vi "lab #5 (displaying cos and sine wave continuously).vi"() -> ()   [LabVIEW 2016]
panel:
  out "Waveform Graph":dynamicdata(graph)
  in  "Phase":dbl
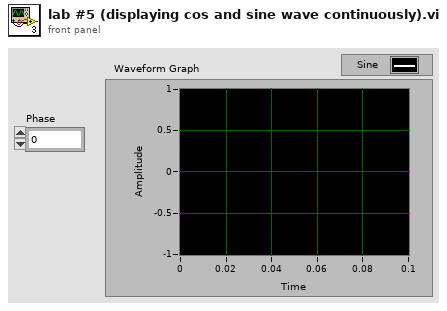
[diagram p1: front panel]
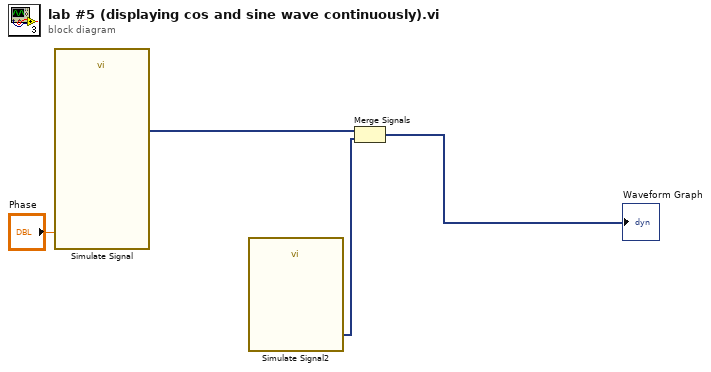
[diagram p0: block diagram]
diagram:
  n1 = call "Simulate Signal"("Phase"="Phase") -> ("Sine"=w4:dynamicdata)  [unwired: 13 in, 1 out]
  n2 = call "Simulate Signal2"() -> ("Sine"=w2:dynamicdata)  [unwired: 14 in, 1 out]
  n3 = Merge Signals(w4, w2) -> (→"Waveform Graph":dynamicdata)
